vi "Core Action.vi"(8 "error in (no error)":errorcluster, 10 "SECS-II Class":refnum<class "SECS-II Class.lvclass">, 11 "07-Event Report From Equipment in":refnum<class "07-Event Report From Equipment.lvclass">) -> (0 "error out":errorcluster, 2 "SECS-II Class Out":refnum<class "SECS-II Class.lvclass">, 3 "07-Event Report From Equipment out":refnum<class "07-Event Report From Equipment.lvclass">)   [LabVIEW 2020, in "SECS Scenarios.lvlib" / "07-Event Report From Equipment.lvclass"]
uses:
  07-Event Report From Equipment.lvclass
  D:/Dropbox/SECS/SECS_GEM v1.1.0/Com/SECS Scenarios/Scenarios Class/Scenarios Class.lvclass
  SECS Communication/SECS-II Class/SECS-II Class.lvclass
  SECS Communication/S6 Message Class/S6 Message Class.lvclass
  D:/Dropbox/SECS/SECS_GEM v1.1.0/Com/SECS Communication/SECS-II Class/SECS-II Class.lvclass
  Scenarios Class/Scenarios Class.lvclass/Scenarios Class.ctl
  Scenarios Class/Reply State.ctl
  Scenarios Class/Write Reply State.vi
  Scenarios Class/Read HSMS Class.vi
  SECS Communication/HSMS Class/HSMS Class.lvclass
  07-Event Report From Equipment.lvclass/07-Event Report From Equipment.ctl
  Scenarios Class/Scenarios Class.lvclass
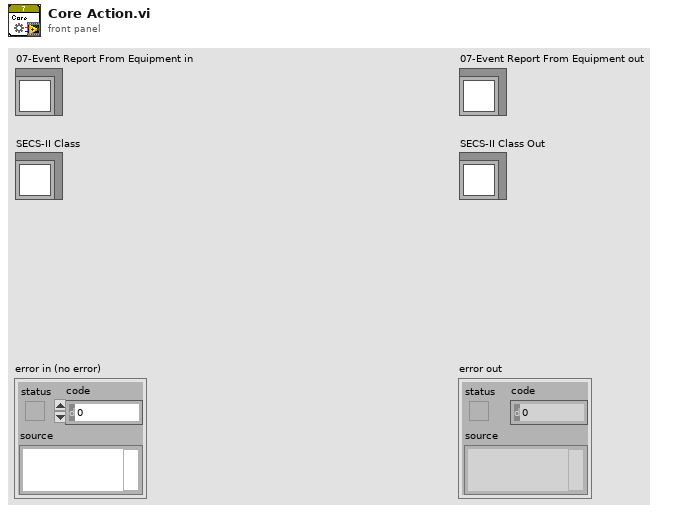
[diagram p1: front panel]
types:
  T1 = typedef "SECS Communication.lvlib/S6 Message Class.lvclass/S6F11.ctl" = cluster{"DATAID":u32, "CEID":u32, "Report Data":cluster{"RPTID":u32, "Value":cluster{"Format Code":T2, "Value":variant}[]}[]}
  T2 = typedef "SECS Communication.lvlib/SECS-II Class.lvclass/Format Code.ctl" = enum16{"L", "A", "B", "Boolean", "J", "I1", "I2", "I4", "I8", "U1", "U2", "U4", "U8", "F4", "F8", "Char"}
  T3 = typedef "SECS Scenarios.lvlib/Scenarios Class.lvclass/Reply State.ctl" = enum16{"OK", "Illegal Data", "Unknown Stream", "Unknown Function", "Off-Line", "T3 Timeout", "Inner-Timeout"}
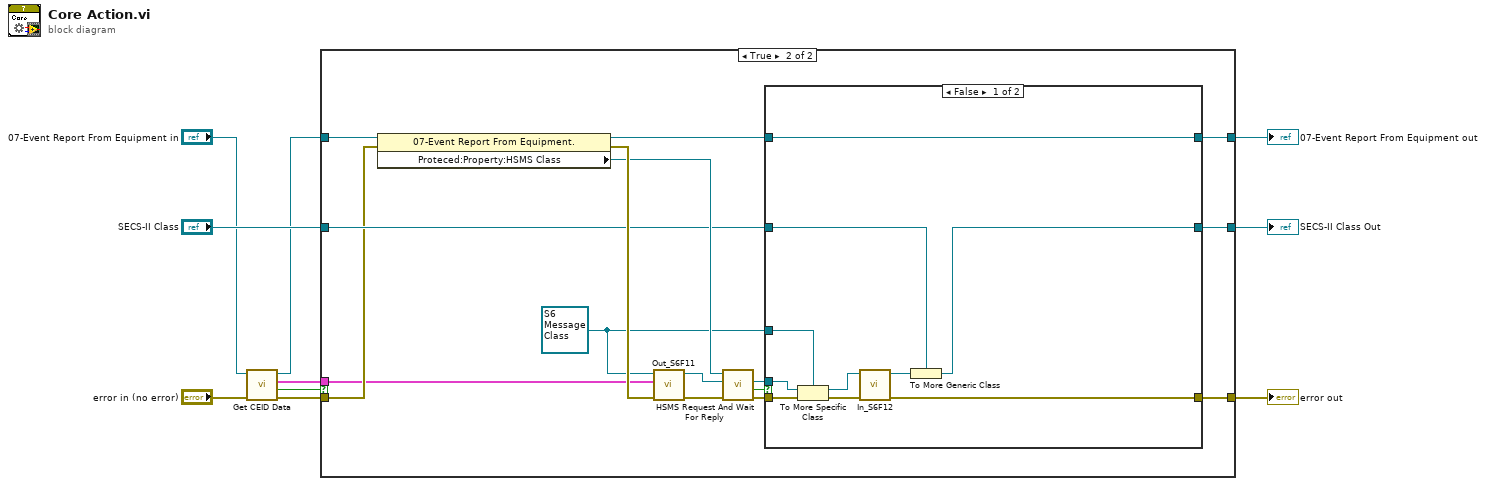
[diagram p0: block diagram]
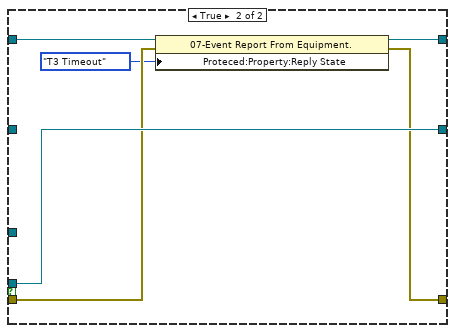
[diagram p3: hidden frame]
diagram:
  n1 = call "Get CEID Data.vi"("error in (no error)"="error in (no error)", "07-Event Report From Equipment in"="07-Event Report From Equipment in") -> ("error out"=w5:errorcluster, "OK?"=w4:bool, "S6F11"=w3:T1, "07-Event Report From Equipment out"=w1:refnum<class "07-Event Report From Equipment.lvclass">)  [unwired: 6 in]
  n2 = case shown="True" w4 {
    tunnel: w5 -> [w12 w15]
    tunnel: w1 -> [w13 w29]
    tunnel: [w13 w20] -> w10
    tunnel: [w12 w23] -> w9
    tunnel: "SECS-II Class" -> [w11 w19]
    tunnel: [w11 w18] -> w7
    tunnel: w3 -> [_ w14]
    frame False {
    }
    frame True {
      w16 = refnum<class "S6 Message Class.lvclass"> refnum ("S6 Message Class in")
      n3 = property class="07-Event Report From Equipment."(reference=w29, error in=w15) -> (reference out=w21:refnum<class "07-Event Report From Equipment.lvclass">, error out=w28:errorcluster, "Proteced:Property:HSMS Class"=w26:refnum<class "HSMS Class.lvclass">)
      n4 = call "Out_S6F11.vi"("error in (no error)"=w28, "S6F11"=w14, "S6 Message Class in"=w16) -> ("error out"=w27:errorcluster, "S6 Message Class out"=w17:refnum<class "S6 Message Class.lvclass">)  [unwired: 7 in]
      n5 = call "HSMS Request And Wait For Reply.vi"("error in (no error)"=w27, "SECS-II Class In"=w17, "HSMS Class in"=w26) -> ("error out"=w25:errorcluster, "Timeout?"=w22:bool, "SECS-II Class Out"=w24:refnum<class "SECS-II Class.lvclass">)  [unwired: 5 in, 1 out]
      n6 = case shown="False" w22 {
        tunnel: w25 -> [w39 w43]
        tunnel: w24 -> [w38 w45]
        tunnel: [w33 w40] -> w23
        tunnel: w21 -> [w35 w44]
        tunnel: [w35 w41] -> w20
        tunnel: w19 -> [w32 _]
        tunnel: [w31 w45] -> w18
        tunnel: w16 -> [w30 _]
        frame False {
          n7 = To More Specific Class(target class=w30, reference=w38, error in=w39) -> (specific class reference=w36:refnum<class "S6 Message Class.lvclass">, error out=w37:errorcluster)
          n8 = call "In_S6F12.vi"("error in (no error)"=w37, "S6 Message Class in"=w36) -> ("error out"=w33:errorcluster, "S6 Message Class out"=w34:refnum<class "S6 Message Class.lvclass">)  [unwired: 6 in, 2 out]
          n9 = To More Generic Class(target class=w32, reference=w34) -> (generic class reference=w31:refnum<class "SECS-II Class.lvclass">)
        }
        frame True {
          n10 = property class="07-Event Report From Equipment."(reference=w44, error in=w43, "Proteced:Property:Reply State"=Reply_State."T3 Timeout" ("Reply State")) -> (reference out=w41:refnum<class "07-Event Report From Equipment.lvclass">, error out=w40:errorcluster)
        }
      }
    }
  }
  "error out" <- w9
  "07-Event Report From Equipment out" <- w10
  "SECS-II Class Out" <- w7
